vi "Read.vi"(8 "error in (no error)":errorcluster, 11 "PCI-4070 in":refnum<class "PCI-4070.lvclass">) -> (0 "error out":errorcluster, 1 "String":string, 2 "Measurement":dbl format="%.5f", 3 "PCI-4070 out":refnum<class "PCI-4070.lvclass">)   [LabVIEW 2012, in "PCI-4070.lvclass"]
uses:
  PCI-4070.lvclass
  DMM Base/DMM.lvclass
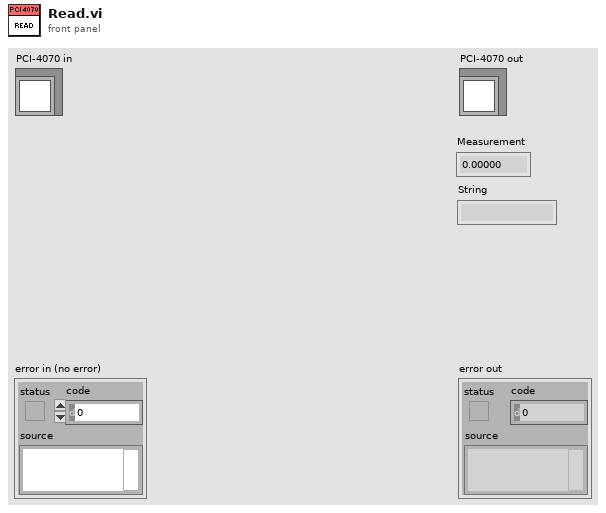
[diagram p1: front panel]
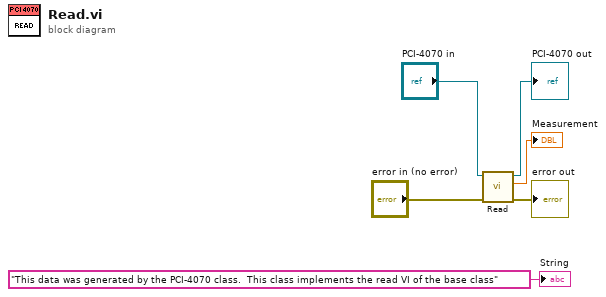
[diagram p0: block diagram]
diagram:
  n1 = call-parent "Read.vi"("error in (no error)"="error in (no error)", "DMM in"="PCI-4070 in") -> ("error out"=→"error out":errorcluster, "Measurement"=→"Measurement":dbl, "DMM out"=→"PCI-4070 out":refnum<class "PCI-4070.lvclass">)  [unwired: 6 in, 1 out]
  "String" <- "This data was generated by the PCI-4070 class.  This class implements the read VI of the base class" ("String")
